vi "SwerveAngleMath.vi"(7 "Turning?":bool, 9 "whRatio":dbl, 10 "Lateral_y":dbl, 11 "Lateral_x":dbl) -> (0 "RRAngle":dbl, 1 "RLAngle":dbl, 2 "FRAngle":dbl, 3 "FLAngle":dbl)   [LabVIEW 2018]
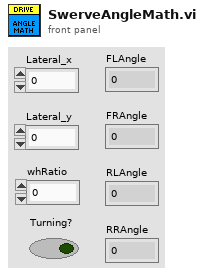
[diagram p1: front panel]
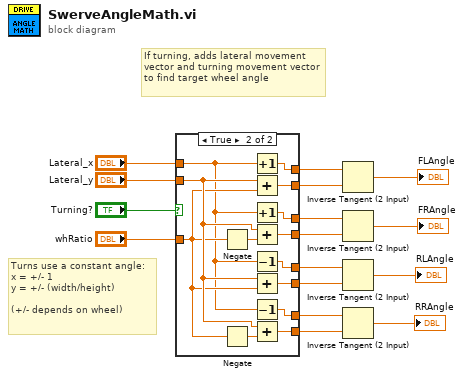
[diagram p0: block diagram]
diagram:
  # "Turns use a constant angle:\nx = +/- 1\ny = +/- (width/height)\n\n(+/- depends on wheel)"
  # "If turning, adds lateral movement vector and turning movement vector to find target wheel angle"
  n1 = case shown="True" "Turning?" {
    tunnel: "Lateral_y" -> [w17 w31]
    tunnel: "whRatio" -> [_ w28]
    tunnel: "Lateral_x" -> [w18 w27]
    tunnel: [w18 w26] -> w13
    tunnel: [w17 w25] -> w12
    tunnel: [w18 w24] -> w11
    tunnel: [w17 w23] -> w10
    tunnel: [w18 w22] -> w9
    tunnel: [w17 w21] -> w8
    tunnel: [w18 w20] -> w7
    tunnel: [w17 w19] -> w6
    frame False {
    }
    frame True {
      n2 = Negate(x=w28) -> (-x=w30:dbl)
      n3 = Negate(x=w28) -> (-x=w29:dbl)
      n4 = Increment(x=w27) -> (x+1=w26:dbl)
      n5 = Add(x=w31, y=w28) -> (x+y=w25:dbl)
      n6 = Increment(x=w27) -> (x+1=w24:dbl)
      n7 = Add(x=w31, y=w30) -> (x+y=w23:dbl)
      n8 = Decrement(x=w27) -> (x-1=w22:dbl)
      n9 = Add(x=w31, y=w28) -> (x+y=w21:dbl)
      n10 = Decrement(x=w27) -> (x-1=w20:dbl)
      n11 = Add(x=w31, y=w29) -> (x+y=w19:dbl)
    }
  }
  n12 = Inverse Tangent (2 Input)(1:w12, 2:w13) -> (0:→"FLAngle":dbl)
  n13 = Inverse Tangent (2 Input)(1:w10, 2:w11) -> (0:→"FRAngle":dbl)
  n14 = Inverse Tangent (2 Input)(1:w8, 2:w9) -> (0:→"RLAngle":dbl)
  n15 = Inverse Tangent (2 Input)(1:w6, 2:w7) -> (0:→"RRAngle":dbl)
